vi "Done.vi"(8 "error in (no error)":errorcluster, 11 "Message Transport Notifier in":refnum<class "Message Transport Notifier.lvclass">) -> (0 "error out":errorcluster, 3 "Message Transport Notifier out":refnum<class "Message Transport Notifier.lvclass">)   [LabVIEW 2016, in "Stream Mediator.lvlib" / "Message Transport Notifier.lvclass"]
doc: "--\nCopyright © 2017 Composed SystemsI All rights reserved.\n\nAuthor: Jon McBee <jon.mcbee@composed.io>\n\nThis library is provided \"AS IS\" ,WITHOUT WARRANTIES OR\nCONDITIONS OF ANY KIND, either express or implied.\n\nComposed Systems -- composed.io\n\nStream 0.0.1.1\nJon McBee - Composed Systems\nCopyright (c) 2017, Composed Systems"
uses:
  <userlib>/Composed Systems/Stream/Mediator/Classes/Message Transport Notifier/Message Transport Notifier.lvclass
  <userlib>/Composed Systems/Stream/Mediator/Classes/Message Transport Notifier/Message Transport Notifier.lvclass/Message Transport Notifier.ctl
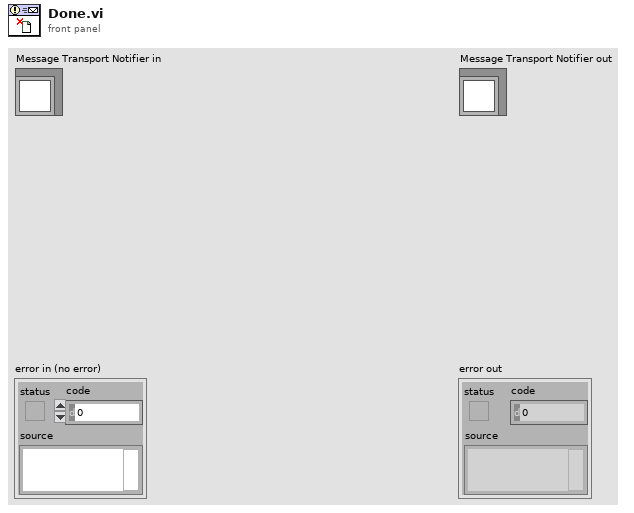
[diagram p1: front panel]
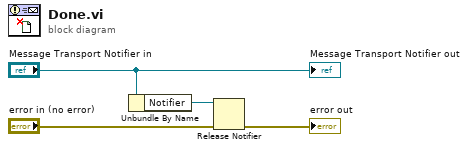
[diagram p0: block diagram]
diagram:
  n1 = Unbundle By Name("Message Transport Notifier in") -> ("Notifier"=w1:refnum<notifier>)
  n2 = Release Notifier(notifier=w1, error in (no error)="error in (no error)") -> (error out=→"error out":errorcluster)  [unwired: 1 in, 2 out]
  "Message Transport Notifier out" <- "Message Transport Notifier in"
